vi "Initialize Gamry.vi"() -> ()   [LabVIEW 2023]
uses:
  TypeDefsControls/Gamry_sensitivity.ctl
  TypeDefsControls/Gamry_Voltagerange.ctl
  TypeDefsControls/Gamry_Pstatmode.ctl
  TypeDefsControls/Gamry_IEstability.ctl
panel:
  in  "Voltage Range":T1 items=["+/- 10 V"=10]
  in  "Sensitivity":T2 items=["60 pA"=1, "600 pA"=2, "6 nA"=3, "60 nA"=4, "600 nA"=5, "6 uA"=6, "60 uA"=7, "600 uA"=8, "6 mA"=9, "60 mA"=10, "600 mA"=11]
  out "error out":errorcluster
  out "Potentiostat Model":string
  in  "GAMRYCOMLib.IGamryPstat":refnum<k7>
  in  "GAMRYCOMLib.IGamryDeviceList":refnum<k7>
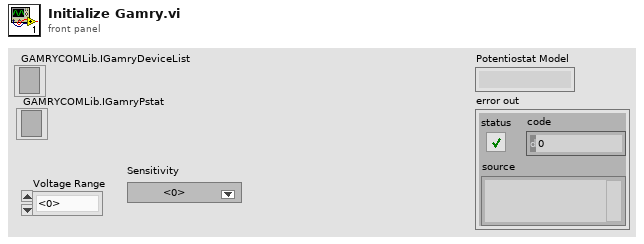
[diagram p1: front panel]
types:
  T1 = typedef "Gamry_Voltagerange.ctl" = u16
  T2 = typedef "Gamry_sensitivity.ctl" = u16
  T3 = typedef "Gamry_IEstability.ctl" = i32
  T4 = typedef "Gamry_Pstatmode.ctl" = i32
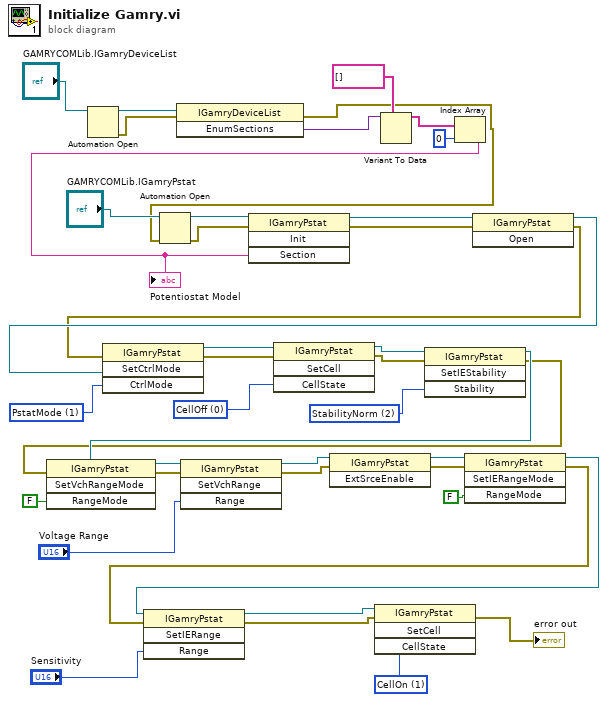
[diagram p0: block diagram]
diagram:
  w13 = T3 2 items=["StabilityFast", "StabilityMedFast", "StabilityNorm", "StabilitySlow"] ("Stability")
  w16 = 0 items=["CellOff", "CellOn", "CellMon", "CellRelay"] ("CellState")
  w19 = T4 1 items=["GstatMode", "PstatMode", "ZRAMode", "FRAMode"] ("CtrlMode")
  w28 = 1 items=["CellOff", "CellOn", "CellMon", "CellRelay"] ("CellState")
  n1 = Automation Open(Automation Refnum="GAMRYCOMLib.IGamryDeviceList") -> (Automation Refnum=w39:refnum<k7>, error out=w38:errorcluster)  [unwired: 3 in]
  n2 = invoke class="IGamryDeviceList" method="EnumSections"(reference=w39, error in=w38) -> (error out=w30:errorcluster, "EnumSections"=w37:variant)  [unwired: 1 in, 1 out]
  n3 = Automation Open(error in (no error)=w30, Automation Refnum="GAMRYCOMLib.IGamryPstat") -> (Automation Refnum=w32:refnum<k7>, error out=w31:errorcluster)  [unwired: 2 in]
  n4 = Variant To Data(type=string[] [], Variant=w37) -> (data=w35:string[])  [unwired: 1 in, 1 out]
  n5 = Index Array(array=w35, index=0) -> (element=w29:string)
  "Potentiostat Model" <- w29
  n6 = invoke class="IGamryPstat" method="Init"(reference=w32, error in=w31, "Section"=w29) -> (reference out=w21:refnum<k7>, error out=w20:errorcluster)  [unwired: 1 in, 2 out]
  n7 = invoke class="IGamryPstat" method="Open"(reference=w21, error in=w20) -> (error out=w1:errorcluster)  [unwired: 1 in, 2 out]
  n8 = invoke class="IGamryPstat" method="SetCtrlMode"(reference=w21, error in=w1, "CtrlMode"=w19) -> (reference out=w18:refnum<k7>, error out=w17:errorcluster)  [unwired: 1 in, 2 out]
  n9 = invoke class="IGamryPstat" method="SetCell"(reference=w18, error in=w17, "CellState"=w16) -> (reference out=w15:refnum<k7>, error out=w14:errorcluster)  [unwired: 1 in, 2 out]
  n10 = invoke class="IGamryPstat" method="SetIEStability"(reference=w15, error in=w14, "Stability"=w13) -> (reference out=w12:refnum<k7>, error out=w11:errorcluster)  [unwired: 1 in, 2 out]
  n11 = invoke class="IGamryPstat" method="SetVchRangeMode"(reference=w12, error in=w11, "RangeMode"=FALSE) -> (reference out=w8:refnum<k7>, error out=w7:errorcluster)  [unwired: 1 in, 2 out]
  n12 = invoke class="IGamryPstat" method="SetVchRange"(reference=w8, error in=w7, "Range"="Voltage Range") -> (reference out=w6:refnum<k7>, error out=w5:errorcluster)  [unwired: 1 in, 2 out]
  n13 = invoke class="IGamryPstat" method="ExtSrceEnable"(reference=w6, error in=w5) -> (reference out=w26:refnum<k7>, error out=w25:errorcluster)  [unwired: 1 in, 1 out]
  n14 = invoke class="IGamryPstat" method="SetIERangeMode"(reference=w26, error in=w25, "RangeMode"=FALSE) -> (reference out=w2:refnum<k7>, error out=w3:errorcluster)  [unwired: 1 in, 2 out]
  n15 = invoke class="IGamryPstat" method="SetIERange"(reference=w2, error in=w3, "Range"="Sensitivity") -> (reference out=w24:refnum<k7>, error out=w23:errorcluster)  [unwired: 1 in, 2 out]
  n16 = invoke class="IGamryPstat" method="SetCell"(reference=w24, error in=w23, "CellState"=w28) -> (error out=→"error out":errorcluster)  [unwired: 1 in, 3 out]
